vi "OpenFileDAQ.vi"(0 "DAQ File Name":string, 3 "error in":errorcluster) -> (7 "appended path":path, 10 "error out":errorcluster)   [LabVIEW 2020, in "DAQ.lvclass"]
uses:
  DAQ/DAQ.lvclass
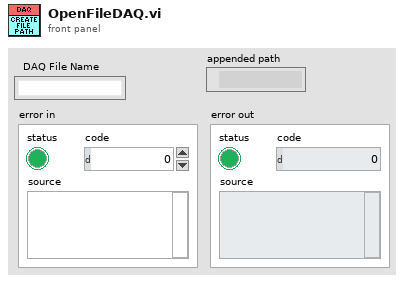
[diagram p1: front panel]
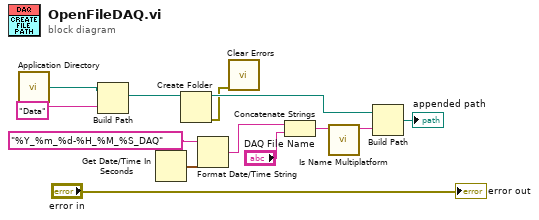
[diagram p0: block diagram]
diagram:
  n1 = call <vilib>:"Application Directory.vi"() -> ("Application Directory"=w10:path)
  n2 = Build Path(base path=w10, name or relative path="Data") -> (appended path=w5:path)
  n3 = Get Date/Time In Seconds() -> (seconds since 1Jan1904=w6:timestamp)
  n4 = Create Folder(path (use dialog)=w5) -> (created path=w4:path, error out=w3:errorcluster)  [unwired: 2 in, 1 out]
  n5 = Format Date/Time String(time format string (%c)="%Y_%m_%d-%H_%M_%S_DAQ", seconds (now)=w6) -> (date/time string=w12:string)  [unwired: 1 in]
  n6 = call <vilib>:"Clear Errors.vi"("error in (no error)"=w3) -> ()  [unwired: 5 in, 2 out]
  n7 = Concatenate Strings(w12, "DAQ File Name") -> (w8:string)
  n8 = call <vilib>:"Is Name Multiplatform.vi"("filename"=w8) -> ("suggested filename"=w7:string)  [unwired: 6 in, 4 out]
  n9 = Build Path(base path=w4, name or relative path=w7) -> (appended path=→"appended path":path)
  "error out" <- "error in"
